vi "Initialize MeasurementLink Session.vi"(7 "remote connection options":T2, 8 "error in":errorcluster, 9 "initialize and close session behavior":T1, 10 "session initialization parameters":T3, 11 "session factory in":refnum<class "NI-DCPower.lvclass">) -> (0 "error out":errorcluster, 2 "session out":variant, 3 "session factory out":refnum<class "NI-DCPower.lvclass">)   [LabVIEW 2020, in "NI-DCPower.lvclass"]
doc: "Creates a new session using the provided <b>session initialization parameters</b>. If the session represents a remote session, <b>initialize and close session behavior</b> determines whether creating the local session creates a new session on the server or attaches to an existing session on the server."
uses:
  NI-DCPower.lvclass
  <vilib>/MeasurementLink/MeasurementLink Instrument/ISession Factory/Session Initialization Parameters.ctl
  <vilib>/MeasurementLink/MeasurementLink Instrument/ISession Factory/Remote Connection Options.ctl
  <vilib>/MeasurementLink/MeasurementLink Instrument/ISession Factory/Initialize and Close Session Behavior.ctl
  NI-DCPower.lvclass/NI-DCPower.ctl
  <vilib>/MeasurementLink/MeasurementLink Instrument/ISession Factory/ISession Factory.lvclass
  <instrlib>/niDCPower/nidcpower.llb/niDCPower Initialize With Independent Channels for gRPC session.vi
  <instrlib>/niDCPower/nidcpower.llb/niDCPower Attach gRPC session.vi
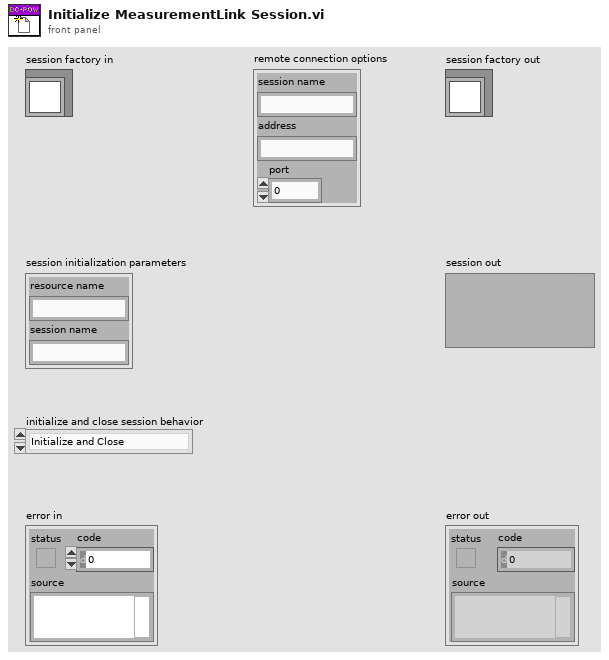
[diagram p1: front panel]
types:
  T1 = typedef "MeasurementLink Instrument.lvlib/ISession Factory.lvclass/Initialize and Close Session Behavior.ctl" = enum16{"Initialize and Close", "Attach and Detach", "Initialize and Detach", "Attach and Close"}
  T2 = typedef "MeasurementLink Instrument.lvlib/ISession Factory.lvclass/Remote Connection Options.ctl" = cluster{"session name":string, "address":string, "port":u32}
  T3 = typedef "MeasurementLink Instrument.lvlib/ISession Factory.lvclass/Session Initialization Parameters.ctl" = cluster{"resource name":string, "session name":string}
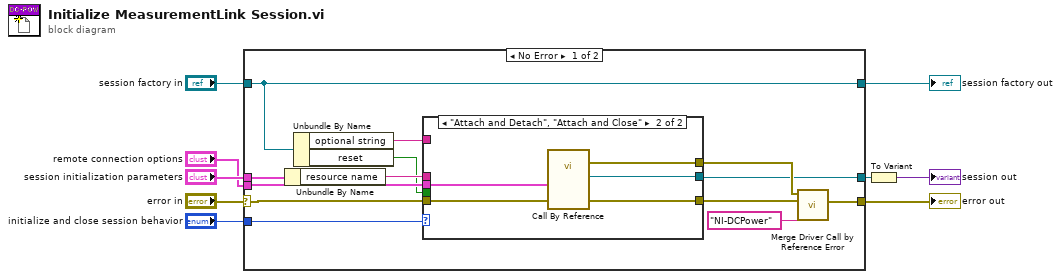
[diagram p0: block diagram]
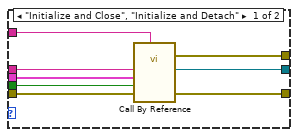
[diagram p2: hidden frame]
diagram:
  n1 = case shown="No Error" "error in" {
    selector: "error in" -> [w18 w36]
    tunnel: [w19 w36] -> w3
    tunnel: "session factory in" -> [w21 w37]
    tunnel: [w21 w37] -> w8
    tunnel: "initialize and close session behavior" -> [w10 _]
    tunnel: "remote connection options" -> [w12 _]
    tunnel: "session initialization parameters" -> [w22 _]
    tunnel: [w15 _] -> w2
    frame No Error {
      n2 = Unbundle By Name(w22) -> ("resource name"=w13:string)
      n3 = Unbundle By Name(w21) -> ("optional string"=w14:string, "reset"=w11:bool)
      n4 = case shown="\"Attach and Detach\", \"Attach and Close\"" w10 {
        tunnel: w12 -> [w29 w35]
        tunnel: [w28 w34] -> w15
        tunnel: w18 -> [w30 w33]
        tunnel: [w24 w32] -> w17
        tunnel: w13 -> [w27 _]
        tunnel: w14 -> [w26 _]
        tunnel: w11 -> [w25 _]
        tunnel: [w23 w31] -> w16
        frame "Initialize and Close", "Initialize and Detach" {
          n5 = call-by-ref "?"("option string"=w26, "error in (no error)"=w30, "reset (false)"=w25, "gRPC options"=w29, "resource name"=w27) -> (error out=w23:errorcluster, 0:"error out"=w24:errorcluster, "instrument handle out"=w28:refnum<k15>)  [unwired: 7 in, 1 out]
        }
        frame "Attach and Detach", "Attach and Close" {
          n6 = call-by-ref "?"("error in (no error)"=w33, "gRPC options"=w35) -> (error out=w31:errorcluster, 0:"error out"=w32:errorcluster, "instrument handle out"=w34:refnum<k15>)  [unwired: 10 in, 1 out]
        }
      }
      n7 = call <vilib>:"Merge Driver Call by Reference Error.vi"("driver name"="NI-DCPower", "called vi error"=w17, "call by ref error"=w16) -> ("error out"=w19:errorcluster)  [unwired: 8 in]
    }
    frame Error {
    }
  }
  "error out" <- w3
  "session factory out" <- w8
  n8 = To Variant(anything=w2) -> (Variant=→"session out":variant)
